vi "Call function.vi"(5 "log file path":string, 6 "cluster of jsons":T1, 7 "night dir":string, 8 "error in (no error)":errorcluster, 9 "Array":u16[][](array[numeric]), 10 "file name":string, 11 "Python Toolkit in":refnum<class "Python Toolkit.lvclass">) -> (0 "error out":errorcluster, 3 "Python Toolkit out":refnum<class "Python Toolkit.lvclass">)   [LabVIEW 2018, in "Python Toolkit.lvclass"]
doc: "Call a python function"
uses:
  Python Toolkit.lvclass
  Python Toolkit.lvclass/Python Toolkit.ctl
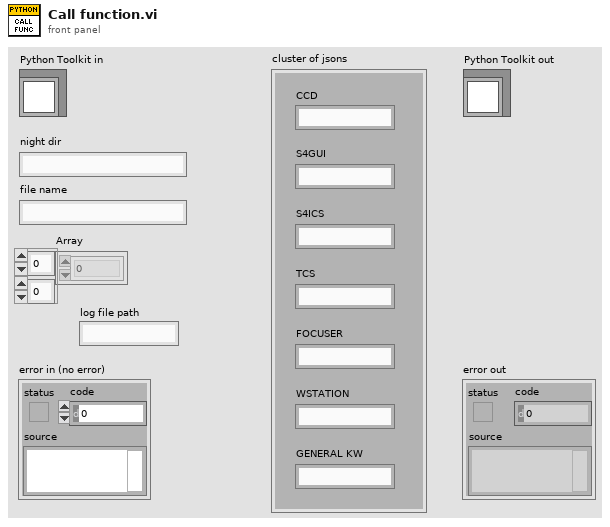
[diagram p1: front panel]
types:
  T1 = cluster{"CCD":string, "S4GUI":string, "S4ICS":string, "TCS":string, "FOCUSER":string, "WSTATION":string, "GENERAL KW":string}
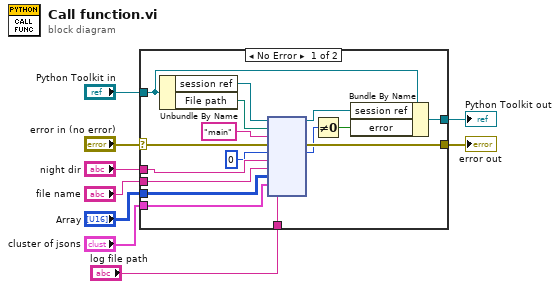
[diagram p0: block diagram]
diagram:
  n1 = case shown="No Error" "error in (no error)" {
    selector: "error in (no error)" -> [w25 w27]
    tunnel: [w24 w27] -> w8
    tunnel: [w22 w26] -> w6
    tunnel: "Python Toolkit in" -> [w23 w26]
    tunnel: "night dir" -> [w17 _]
    tunnel: "file name" -> [w16 _]
    tunnel: "Array" -> [w15 _]
    tunnel: "cluster of jsons" -> [w11 _]
    tunnel: "log file path" -> [w10 _]
    frame No Error {
      n2 = Unbundle By Name(w23) -> ("session ref"=w20:refnum<k35>, "File path"=w19:path)
      n3 = node(w20, w19, "main" ("function name"), w25, u8 0, w17, w16, w15, w11, w10) -> (w21:refnum<k35>, w24:errorcluster, w13:u8)  [unwired: 5 in, 2 out]
      n4 = Not Equal To 0?(x=w13) -> (x != 0?=w12:bool)
      n5 = Bundle By Name(cluster=w23, "session ref"=w21, "error"=w12) -> (w22:refnum<class "Python Toolkit.lvclass">)
    }
    frame Error {
    }
  }
  "error out" <- w8
  "Python Toolkit out" <- w6
